vi "温度校准读取.vi"(8 "Error in":errorcluster caption="Error in (no error)", 11 "站号":u16(ring)=10 items=["氨氮"=3, "水温"=9, "pH值"=10, "溶解氧"=11, "电导率"=12, "浊度"=13, "叶绿素a"=14, "藻密度"=15, "蓝绿藻"=16, "氧化还原电位"=17, "溶解氧%"=18, "盐度"=19]) -> (0 "error out":errorcluster, 2 "Bt":sgl, 3 "Kt":sgl)   [LabVIEW 2016, in "斯坦道原位多参数.lvlib"]
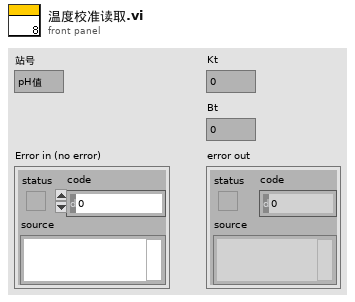
[diagram p1: front panel]
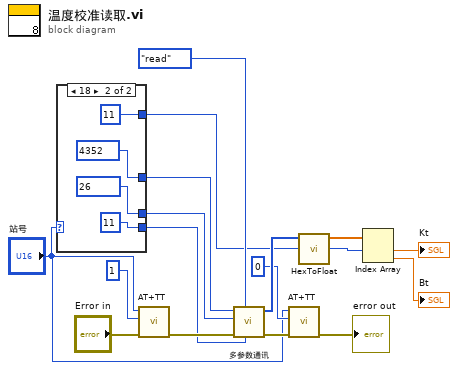
[diagram p0: block diagram]
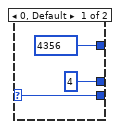
[diagram p2: hidden frame]
diagram:
  n1 = case shown="18" "站号" {
    selector: "站号" -> [w19 _]
    tunnel: [w19 u16 11 ("站号")] -> w9
    tunnel: [u16 4356 ("starting address") u16 4352 ("starting address")] -> w4
    tunnel: [u16 4 ("quantity") u16 26 ("starting address")] -> w2
    tunnel: [_ 11 ("索引")] -> w1
    frame 0, Default {
    }
    frame 18 {
    }
  }
  n2 = call "AT+TT.vi"("错误输入（无错误）"="Error in", "Count"=1, "站号"="站号") -> ("错误输出"=w12:errorcluster)  [unwired: 7 in, 1 out]
  n3 = call "多参数通讯.vi"("Slave ID"=w9, "STEP"=enum16{"open", "read", "write", "close"}."read", "Error in"=w12, "quantity"=w2, "starting address"=w4) -> ("error out"=w8:errorcluster, "Registers"=w16:u16[])  [unwired: 4 in, 1 out]
  n4 = call "AT+TT.vi"("错误输入（无错误）"=w8, "Count"=0, "站号"="站号") -> ("错误输出"=→"error out":errorcluster)  [unwired: 7 in, 1 out]
  n5 = call "HexToFloat.vi"("数组"=w16) -> ("FLOAT"=w15:sgl[])  [unwired: 10 in]
  n6 = Index Array(array=w15, index #1=w1) -> (element #1=→"Kt":sgl, element #2=→"Bt":sgl)  [unwired: 1 in]
